vi "高压板校正命令.vi"(0 "CAN卡类型":u32(ring)=4 items=["PCI5121"=1, "PCI9810"=2, "USBCAN1"=3, "USBCAN2"=4, "PCI9820"=5, "PCI5110"=7, "CANLite(mini)"=8, "ISA9620"=9, "ISA5420"=10, "PC104CAN"=11, "DNP9810"=13, "PCI9840B"=14, "PC104C2"=15, "PCI9820I"=16, "pec9920"=18, "USBCAN_E_U"=20, "USBCAN_2E_U"=21], 1 "设备索引":u16(ring) items=["0", "1", "2", "3", "4", "5", "6", "7", "8", "9", "10", "11", "12", "13", "14", "15", ""], 2 "波特率":T4(ring)=enum."250Kbps", 3 "CAN路数":u16(ring) items=["0", "1"], 4 "Data Input":string, 5 "error in (no error)":errorcluster caption="错误输入（无错误）", 6 "滤波方式":u8(ring)=1 items=["Dual Filter", "Single Filter"], 8 "传入类型":enum16{"ASCII字符", "16进制字符"}(ring), 10 "工作方式":u8(ring) items=["Normal", "Listen Only"], 11 "校准命令":T3(ring)) -> (14 "结果":bool=TRUE, 15 "VCI_CAN_OBJ_R":T2={"ID"=0, "TimeStamp"=0, "TimeFlag"=0, "SendType"=1, "RemoteFlag"=0, "ExternFlag"=0, "DataLen"=8, 0, 0, 0, 0, 0, 0, 0, 0, 0, 0, 0} {"ID" format="%x"}, 16 "添加的数组":u8[](array[numeric]), 19 "错误输出":errorcluster)   [LabVIEW 2013]
uses:
  data/ControlCAN.dll
panel:
  out "E-U_baud":u32(ring)=393223 items=["0x060003--1000Kbps"=393219, "0x060004--800Kbps"=393220, "0x060007--500Kbps"=393223, "0x1C0008--250Kbps"=1835016, "0x1C0011--125Kbps"=1835025, "0x160023--100Kbps"=1441827, "0x1C002C--50Kbps"=1835052, "0x1600B3--20Kbps"=1441971, "0x1C00E0--10Kbps"=1835232, "0x1C01C1--5Kbps"=1835457]
  in  "等待时间（毫秒）":u32=500
  in  "times":dbl
  out "簇":T1
  out "输出簇":T2 {"ID" format="%x"}
  out "VCI_CAN_OBJ_T 2":T2
  out "子字符串":string
  in  "期望字符串":string
  in  "长度":i32
  out "VCI_CAN_OBJ_T":T2 {"ID" format="%x"}
  in  "DeviceType 5":u16(ring)=1 items=["PCI5121"=1, "PCI9810"=2, "USBCAN1"=3, "USBCAN2"=4, "PCI9820"=5, "CAN232"=6, "PCI5110"=7, "CANLite(mini)"=8, "ISA9620"=9, "ISA5420"=10, "PC104CAN"=11, "CANETE"=12, "DNP9810"=13]
  in  "CAN Channel 3":u16(ring) items=["0", "1"]
  in  "DeviceType 4":u16(ring)=1 items=["PCI5121"=1, "PCI9810"=2, "USBCAN1"=3, "USBCAN2"=4, "PCI9820"=5, "CAN232"=6, "PCI5110"=7, "CANLite(mini)"=8, "ISA9620"=9, "ISA5420"=10, "PC104CAN"=11, "CANETE"=12, "DNP9810"=13]
  in  "Accept Code":u32 format="%08x"
  in  "Mask Code":u32=4294967295 format="%08x"
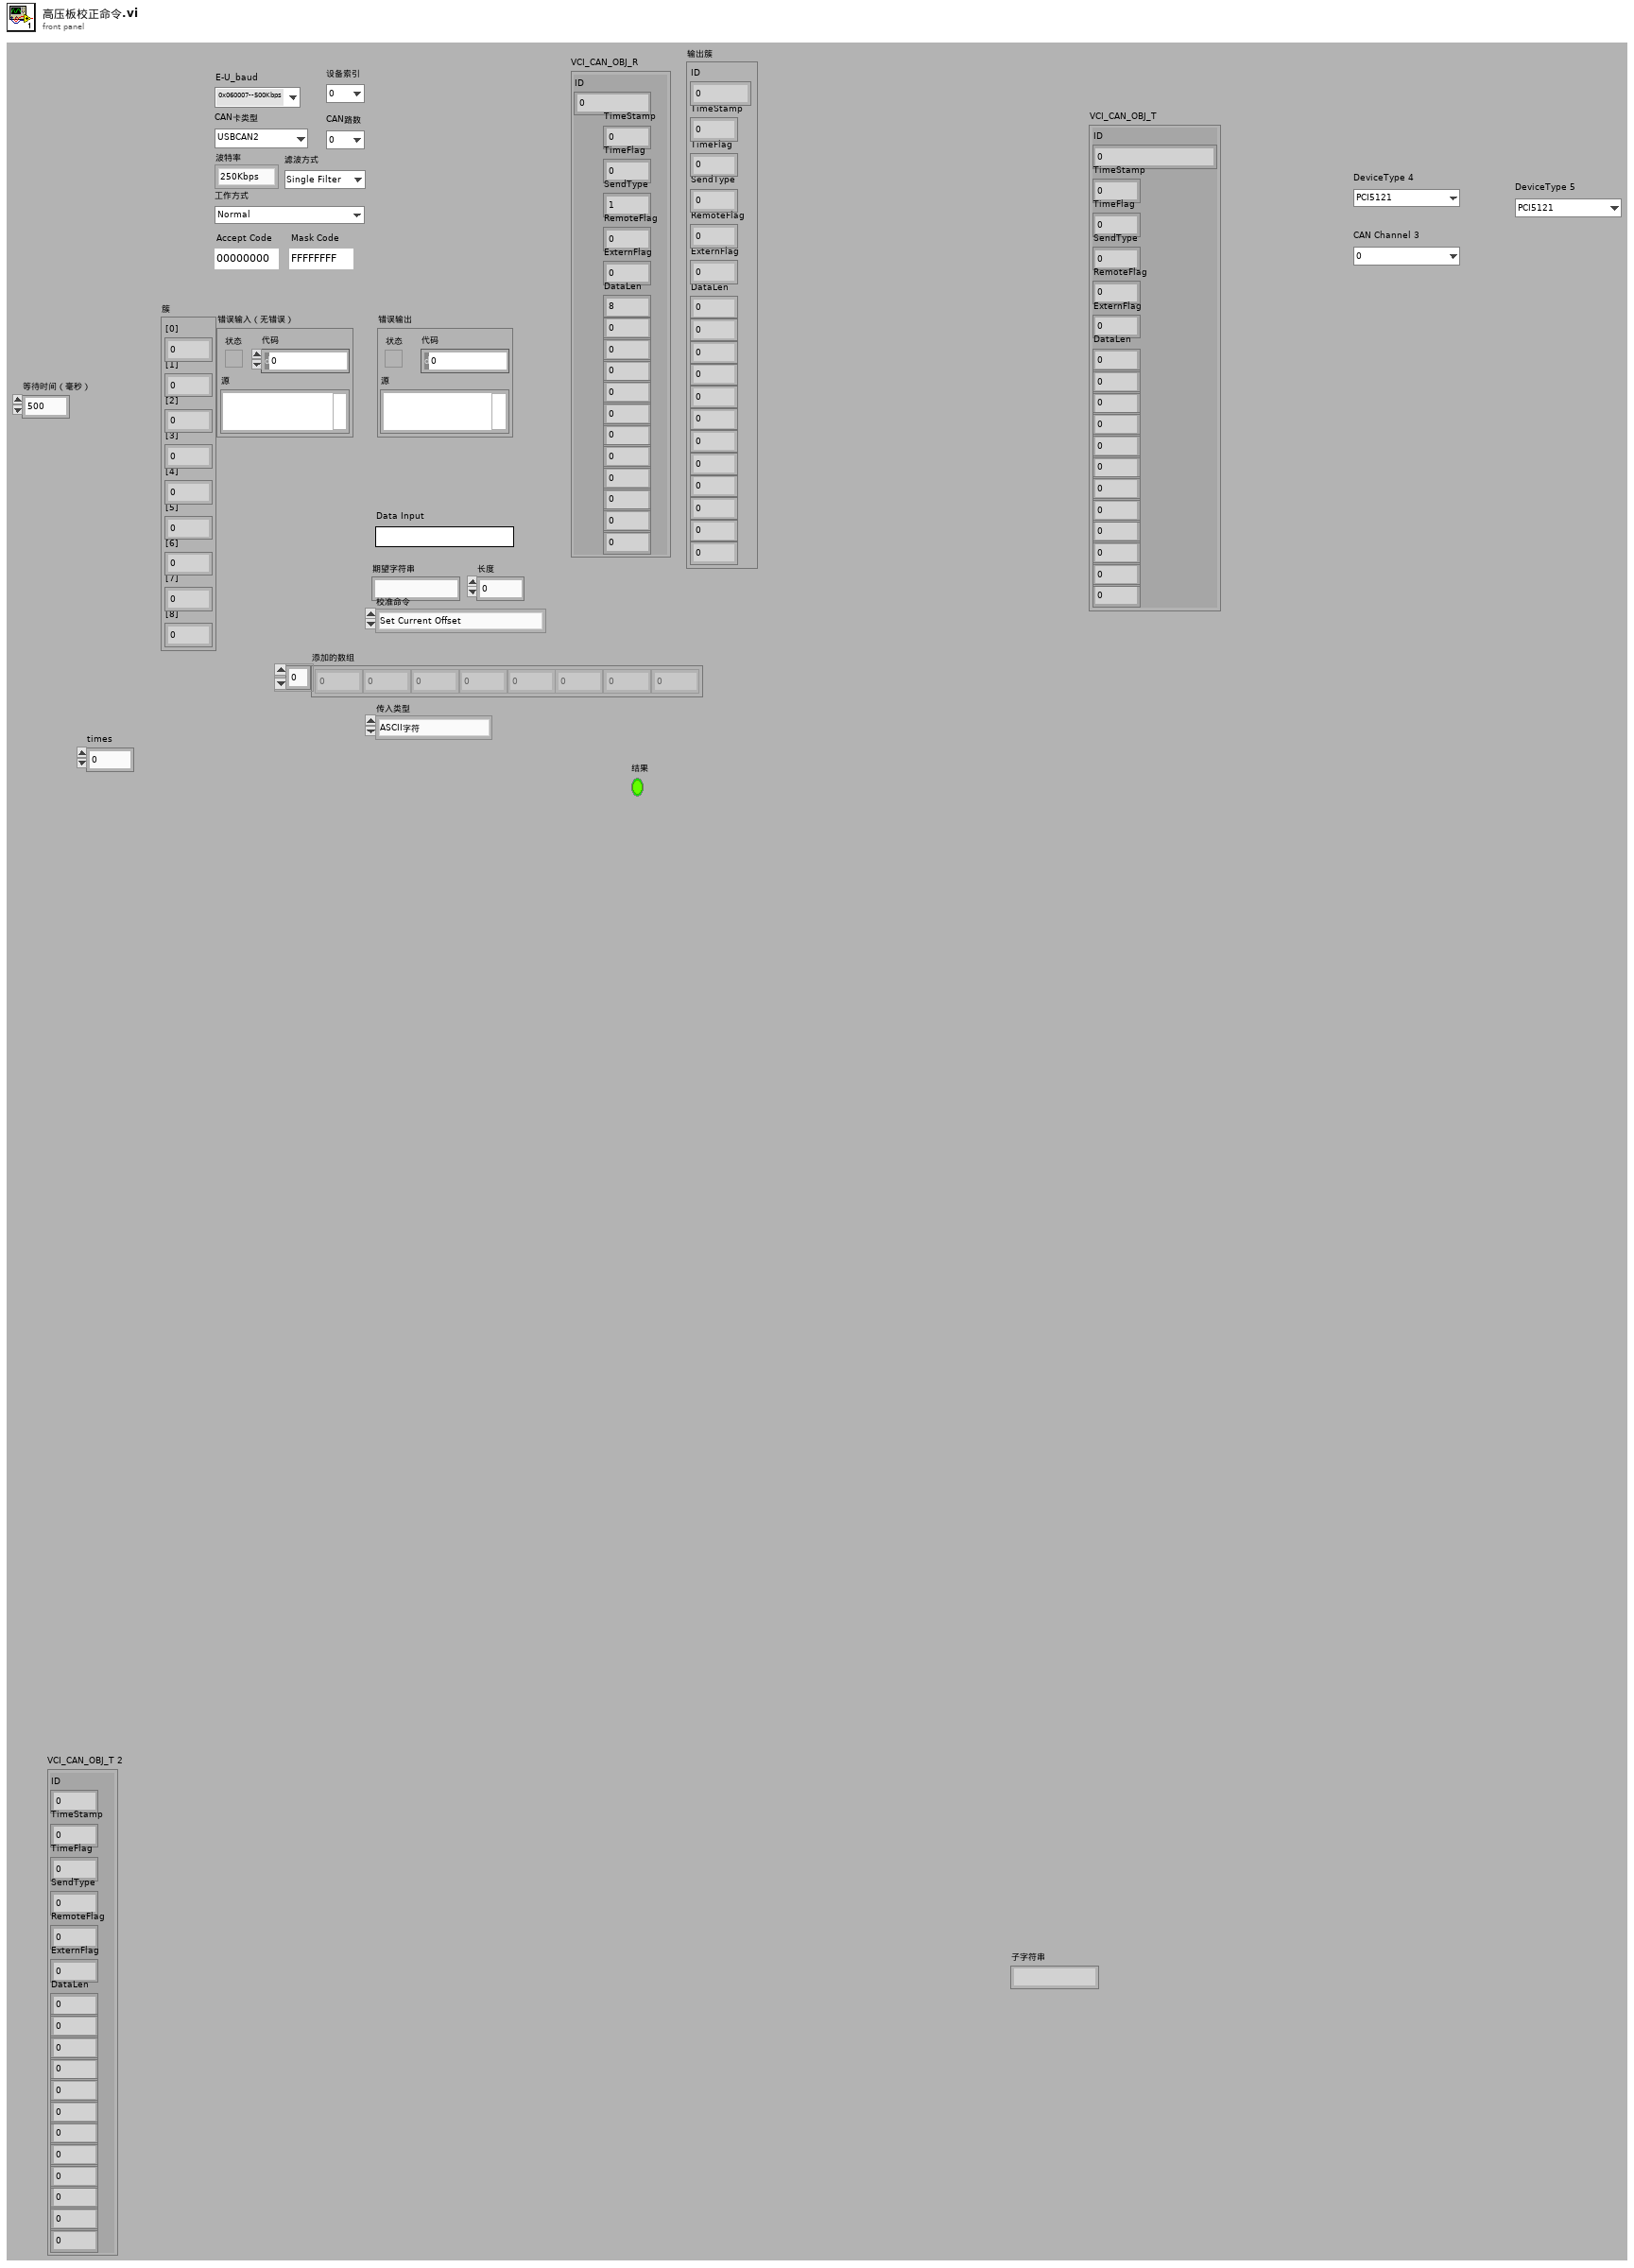
[diagram p1: front panel]
types:
  T1 = cluster{"[0]":i32, "[1]":i32, "[2]":i32, "[3]":i32, "[4]":i32, "[5]":i32, "[6]":i32, "[7]":i32, "[8]":i32}
  T2 = cluster{"ID":u32, "TimeStamp":u32, "TimeFlag":u8, "SendType":u8, "RemoteFlag":u8, "ExternFlag":u8, "DataLen":u8, u8, u8, u8, u8, u8, u8, u8, u8, u8, u8, u8}
  T3 = enum16{"Set Current Offset", "Set Current Gain 4", "Set Current Gain", "Set Volt offset", "Set Volt Gain", "Set Current Offset 3", "Set Current Gain 3", "Set Current Offset 4", "Read", "Set", "Clear", "Read_in", "Set_in", "Clear_in", "Read_out", "Set_out", "Clear_out", "参数设置", "写配置文件版本", "读配置文件版本"}
  T4 = enum16{"5Kbps", "10Kbps", "20Kbps", "40Kbps", "50Kbps", "80Kbps", "100Kbps", "125Kbps", "200Kbps", "250Kbps", "400Kbps", "500Kbps", "666Kbps", "800Kbps", "1000Kbps"}
  T5 = cluster{"[0]":u32, "[1]":u32, "[2]":u32, "[3]":u32, "[4]":u32, "[5]":u32, "[6]":u32, "[7]":u32, "[8]":u32}
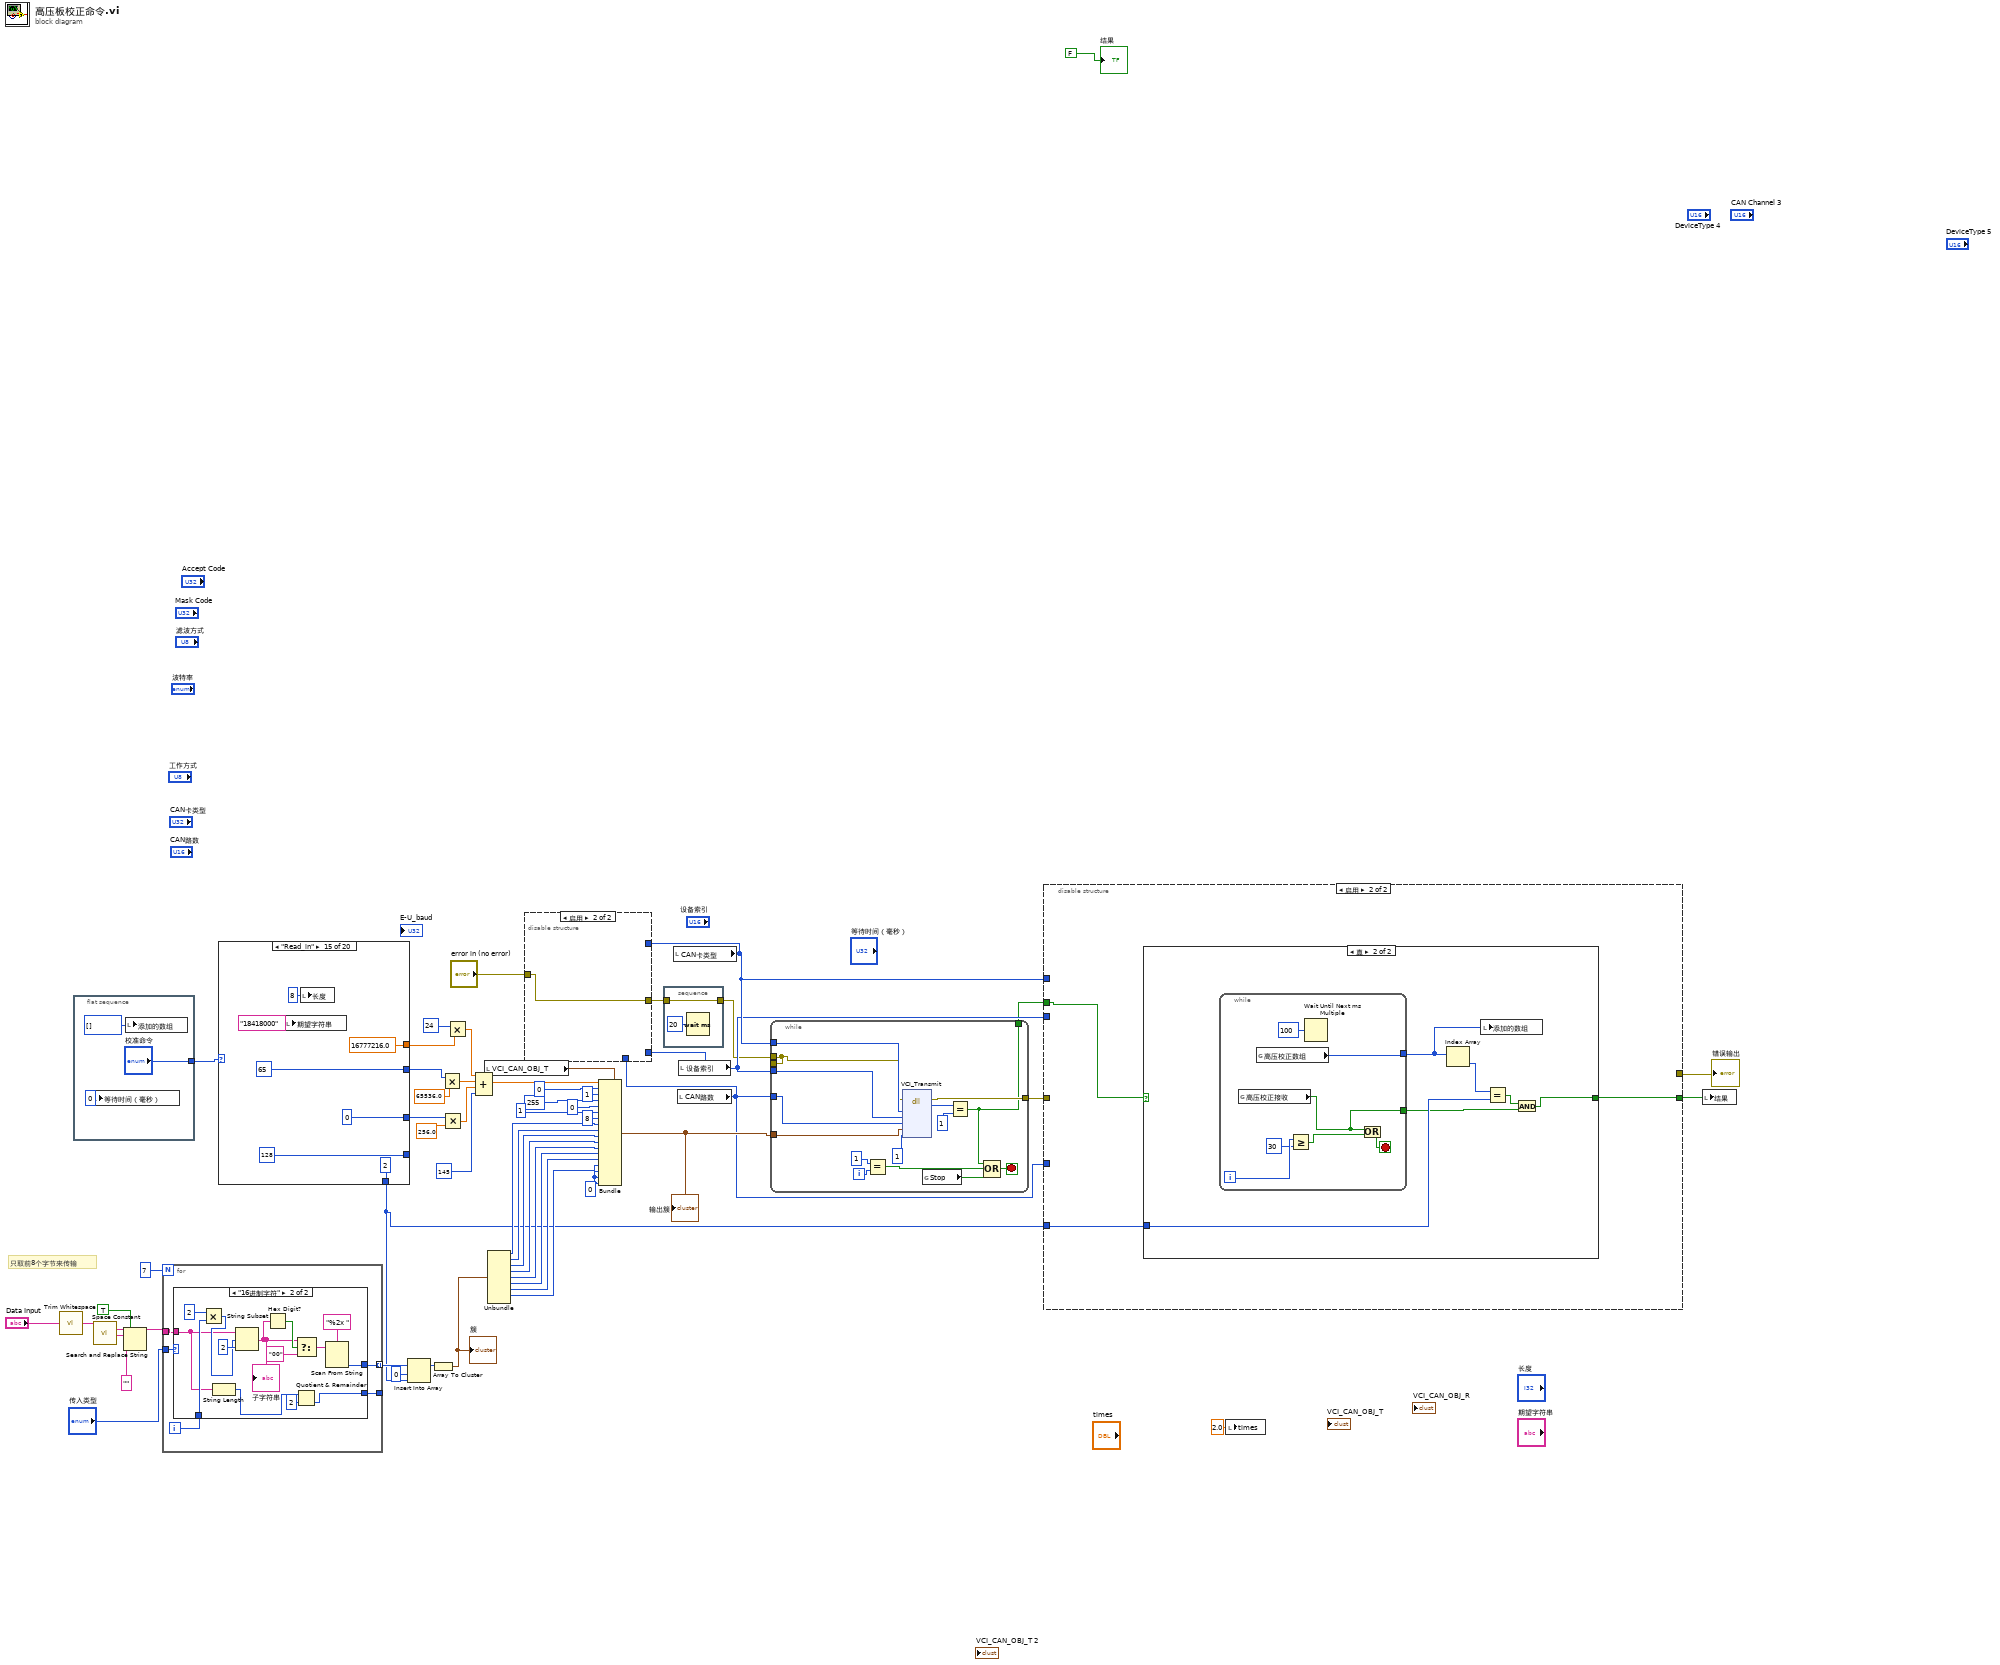
[diagram p0: block diagram]
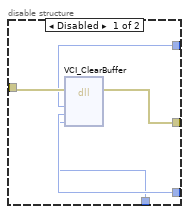
[diagram p2: hidden frame]
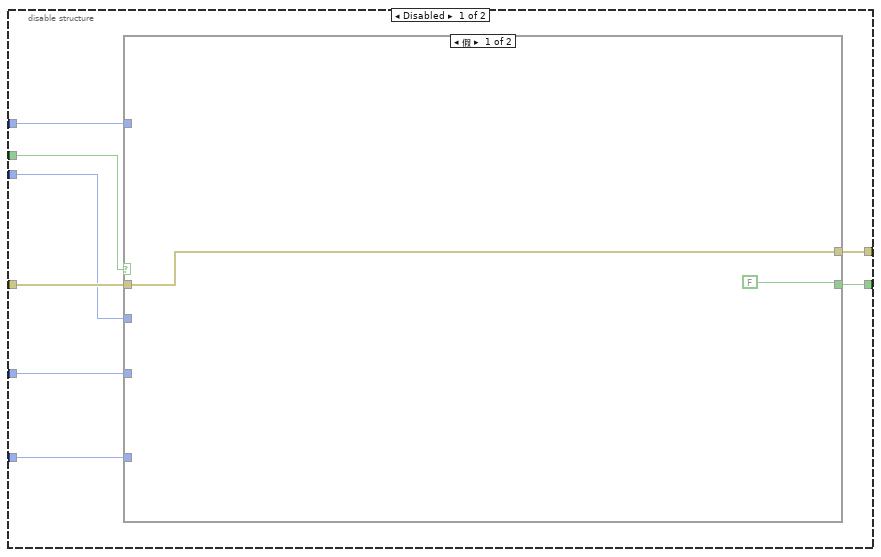
[diagram p3: hidden frame]
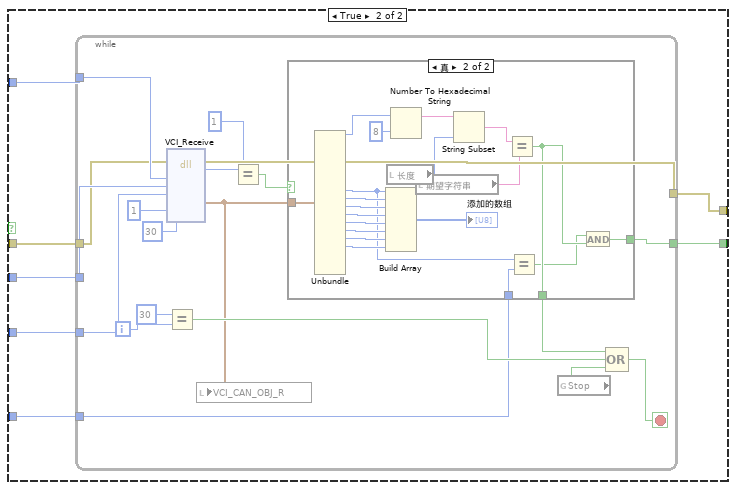
[diagram p4: hidden frame]
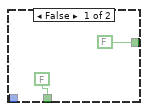
[diagram p5: hidden frame]
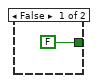
[diagram p6: hidden frame]
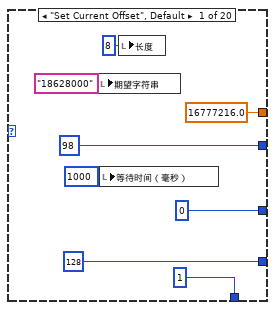
[diagram p7: hidden frame]
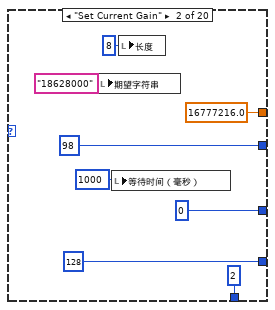
[diagram p8: hidden frame]
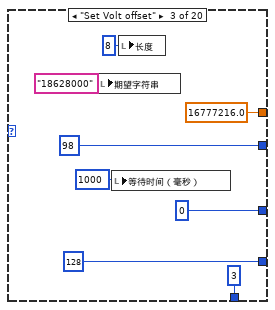
[diagram p9: hidden frame]
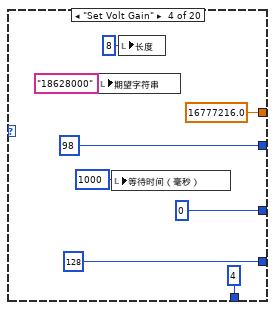
[diagram p10: hidden frame]
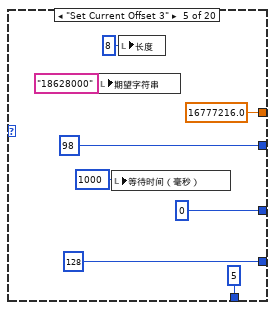
[diagram p11: hidden frame]
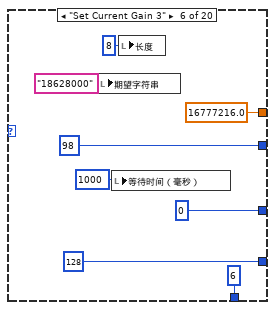
[diagram p12: hidden frame]
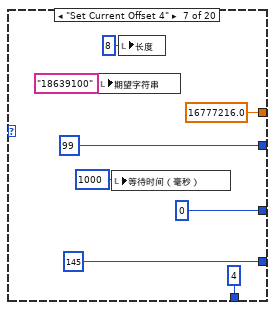
[diagram p13: hidden frame]
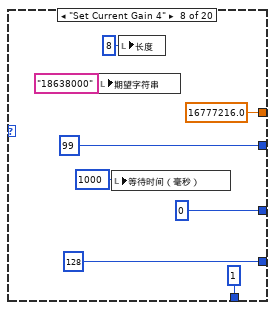
[diagram p14: hidden frame]
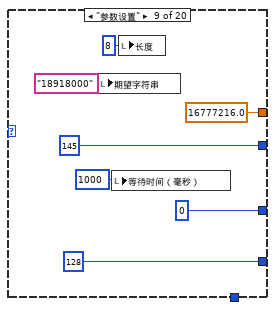
[diagram p15: hidden frame]
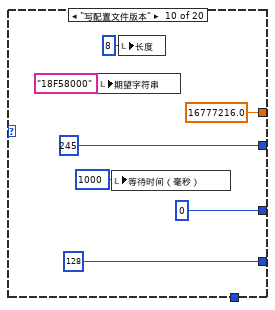
[diagram p16: hidden frame]
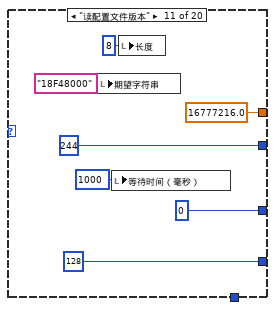
[diagram p17: hidden frame]
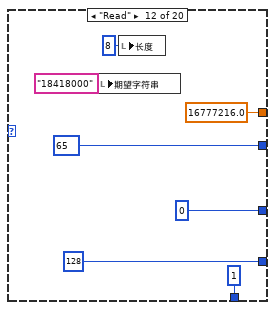
[diagram p18: hidden frame]
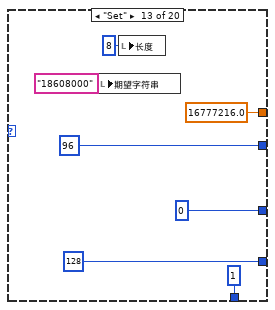
[diagram p19: hidden frame]
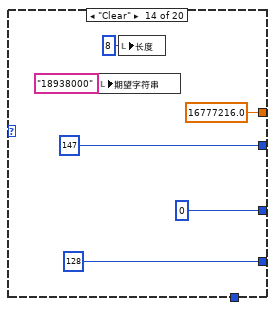
[diagram p20: hidden frame]
diagram:
  w31 = u8 0 ("元素")
  # "只取前8个字节来传输"
  n1 = call <vilib>:"Trim Whitespace.vi"("string"="Data Input") -> ("trimmed string"=w49:string)  [unwired: 1 in]
  n2 = flat-sequence {
    tunnel: ["校准命令"] -> w6
    frame #0 {
      n3 = local write "等待时间（毫秒）"(u32 0 ("等待时间（毫秒）")) -> ()
      n4 = local write "添加的数组"(u8[] [] ("添加的数组")) -> ()
    }
  }
  n5 = call <vilib>:"Space Constant.vi"() -> ("String"=w48:string)
  n6 = Search and Replace String(replace all?=TRUE ("替换全部？(F)"), input string=w49, search string=w48, replace string="" ("替换字符串(\"\")")) -> (result string=w45:string)  [unwired: 1 in, 6 out]
  n7 = for {
    N: 7 -> [_]
    tunnel: w45 -> [w60]
    tunnel: [w62] -> w53 mode=indexing
    tunnel: [w59] -> _
    tunnel: "传入类型" -> [w58]
    i -> [w61]
    n8 = case shown="\"16进制字符\"" w58 {
      tunnel: [w63 w79] -> w62
      tunnel: w61 -> [w66 w74]
      tunnel: w60 -> [w68 w72]
      tunnel: [_ w69] -> w59
      frame "ASCII字符", Default {
        n9 = String Subset(string=w68, offset (0)=w66, length (rest)=1 ("长度（剩余）")) -> (substring=w64:string)
        n10 = Type Cast(type=u8 0, x=w64) -> (*(type *) &x=w63:u8)
      }
      frame "16进制字符" {
        n11 = Multiply(x=2, y=w74) -> (x*y=w73:i32)
        n12 = String Length(string=w72) -> (length=w71:i32)
        n13 = String Subset(string=w72, offset (0)=w73, length (rest)=2 ("length (rest)")) -> (substring=w76:string)
        "子字符串" <- w76
        n14 = Hex Digit?(1:w76) -> (0:w77:bool)
        n15 = Select(t=w76, s=w77, f="00" ("t")) -> (s? t:f=w78:string)
        n16 = Quotient & Remainder(x=w71, y=2) -> (floor(x/y)=w69:i32)  [unwired: 1 out]
        n17 = Scan From String(format string="%2x ", input string=w78) -> (output 1=w79:u32)  [unwired: 2 in, 4 out]
      }
    }
  }
  n18 = case shown="\"Read_in\"" w6 {
    tunnel: [16777216.0 ("y") 16777216.0 ("y") 16777216.0 ("y") 16777216.0 ("y") 16777216.0 ("y") 16777216.0 ("y") 16777216.0 ("y") 16777216.0 ("y") 16777216.0 ("y") 16777216.0 ("y") 16777216.0 ("y") 16777216.0 ("y") 16777216.0 ("y") 16777216.0 ("y") 16777216.0 ("y") 16777216.0 ("y") 16777216.0 ("y") 16777216.0 ("y") 16777216.0 ("y") 16777216.0 ("y")] -> w43
    tunnel: [u32 98 ("x") u32 98 ("x") u32 98 ("x") u32 98 ("x") u32 98 ("x") u32 98 ("x") u32 99 ("x") u32 99 ("x") u32 145 ("x") u32 245 ("x") u32 244 ("x") u32 65 ("x") u32 96 ("x") u32 147 ("x") u32 65 ("x") u32 96 ("x") u32 149 ("x") u32 65 ("x") u32 96 ("x") u32 151 ("x")] -> w39
    tunnel: [u32 0 ("从板号") u32 0 ("从板号") u32 0 ("从板号") u32 0 ("从板号") u32 0 ("从板号") u32 0 ("从板号") u32 0 ("从板号") u32 0 ("从板号") u32 0 ("从板号") u32 0 ("从板号") u32 0 ("从板号") u32 0 ("从板号") u32 0 ("从板号") u32 0 ("从板号") u32 0 ("从板号") u32 0 ("从板号") u32 0 ("从板号") u32 0 ("从板号") u32 0 ("从板号") u32 0 ("从板号")] -> w36
    tunnel: [u32 128 ("x") u32 128 ("x") u32 128 ("x") u32 128 ("x") u32 128 ("x") u32 128 ("x") u32 145 ("x") u32 128 ("x") u32 128 ("x") u32 128 ("x") u32 128 ("x") u32 128 ("x") u32 128 ("x") u32 128 ("x") u32 128 ("x") u32 128 ("x") u32 128 ("x") u32 128 ("x") u32 128 ("x") u32 128 ("x")] -> _
    tunnel: [u32 1 ("从板号") u32 2 ("从板号") u32 3 ("从板号") u32 4 ("从板号") u32 5 ("从板号") u32 6 ("从板号") u32 4 ("从板号") u32 1 ("从板号") _ _ _ u32 1 ("从板号") u32 1 ("从板号") _ u32 2 ("从板号") u32 2 ("从板号") _ u32 3 ("从板号") u32 3 ("从板号") _] -> w3
    frame "Set Current Offset", Default {
      n19 = local write "期望字符串"("18628000" ("期望字符串")) -> ()
      n20 = local write "等待时间（毫秒）"(u32 1000 ("等待时间（毫秒）")) -> ()
      n21 = local write "长度"(8 ("长度")) -> ()
    }
    frame "Set Current Gain" {
      n22 = local write "期望字符串"("18628000" ("期望字符串")) -> ()
      n23 = local write "等待时间（毫秒）"(u32 1000 ("等待时间（毫秒）")) -> ()
      n24 = local write "长度"(8 ("长度")) -> ()
    }
    frame "Set Volt offset" {
      n25 = local write "期望字符串"("18628000" ("期望字符串")) -> ()
      n26 = local write "等待时间（毫秒）"(u32 1000 ("等待时间（毫秒）")) -> ()
      n27 = local write "长度"(8 ("长度")) -> ()
    }
    frame "Set Volt Gain" {
      n28 = local write "期望字符串"("18628000" ("期望字符串")) -> ()
      n29 = local write "等待时间（毫秒）"(u32 1000 ("等待时间（毫秒）")) -> ()
      n30 = local write "长度"(8 ("长度")) -> ()
    }
    frame "Set Current Offset 3" {
      n31 = local write "期望字符串"("18628000" ("期望字符串")) -> ()
      n32 = local write "等待时间（毫秒）"(u32 1000 ("等待时间（毫秒）")) -> ()
      n33 = local write "长度"(8 ("长度")) -> ()
    }
    frame "Set Current Gain 3" {
      n34 = local write "期望字符串"("18628000" ("期望字符串")) -> ()
      n35 = local write "等待时间（毫秒）"(u32 1000 ("等待时间（毫秒）")) -> ()
      n36 = local write "长度"(8 ("长度")) -> ()
    }
    frame "Set Current Offset 4" {
      n37 = local write "期望字符串"("18639100" ("期望字符串")) -> ()
      n38 = local write "等待时间（毫秒）"(u32 1000 ("等待时间（毫秒）")) -> ()
      n39 = local write "长度"(8 ("长度")) -> ()
    }
    frame "Set Current Gain 4" {
      n40 = local write "期望字符串"("18638000" ("期望字符串")) -> ()
      n41 = local write "等待时间（毫秒）"(u32 1000 ("等待时间（毫秒）")) -> ()
      n42 = local write "长度"(8 ("长度")) -> ()
    }
    frame "参数设置" {
      n43 = local write "期望字符串"("18918000" ("期望字符串")) -> ()
      n44 = local write "等待时间（毫秒）"(u32 1000 ("等待时间（毫秒）")) -> ()
      n45 = local write "长度"(8 ("长度")) -> ()
    }
    frame "写配置文件版本" {
      n46 = local write "期望字符串"("18F58000" ("期望字符串")) -> ()
      n47 = local write "等待时间（毫秒）"(u32 1000 ("等待时间（毫秒）")) -> ()
      n48 = local write "长度"(8 ("长度")) -> ()
    }
    frame "读配置文件版本" {
      n49 = local write "期望字符串"("18F48000" ("期望字符串")) -> ()
      n50 = local write "等待时间（毫秒）"(u32 1000 ("等待时间（毫秒）")) -> ()
      n51 = local write "长度"(8 ("长度")) -> ()
    }
    frame "Read" {
      n52 = local write "期望字符串"("18418000" ("期望字符串")) -> ()
      n53 = local write "长度"(8 ("长度")) -> ()
    }
    frame "Set" {
      n54 = local write "期望字符串"("18608000" ("期望字符串")) -> ()
      n55 = local write "长度"(8 ("长度")) -> ()
    }
    frame "Clear" {
      n56 = local write "期望字符串"("18938000" ("期望字符串")) -> ()
      n57 = local write "长度"(8 ("长度")) -> ()
    }
    frame "Read_in" {
      n58 = local write "期望字符串"("18418000" ("期望字符串")) -> ()
      n59 = local write "长度"(8 ("长度")) -> ()
    }
    frame "Set_in" {
      (unwired) u32 4 ("从板号")
      n60 = local write "期望字符串"("18608000" ("期望字符串")) -> ()
      n61 = local write "长度"(8 ("长度")) -> ()
    }
    frame "Clear_in" {
      n62 = local write "期望字符串"("18958000" ("期望字符串")) -> ()
      n63 = local write "长度"(8 ("长度")) -> ()
    }
    frame "Read_out" {
      n64 = local write "期望字符串"("18418000" ("期望字符串")) -> ()
      n65 = local write "长度"(8 ("长度")) -> ()
    }
    frame "Set_out" {
      n66 = local write "期望字符串"("18608000" ("期望字符串")) -> ()
      n67 = local write "长度"(8 ("长度")) -> ()
    }
    frame "Clear_out" {
      n68 = local write "期望字符串"("18978000" ("期望字符串")) -> ()
      n69 = local write "长度"(8 ("长度")) -> ()
    }
  }
  n70 = Insert Into Array(array=w53, index=0 ("索引"), new element=w3) -> (w5:u32[])
  n71 = Array To Cluster(array=w5) -> (cluster=w52:T5)
  "簇" <- w52
  n72 = Multiply(x=w39, y=65536.0) -> (x*y=w38:dbl)
  n73 = Multiply(x=w36, y=256.0) -> (x*y=w35:dbl)
  n74 = Multiply(x=u32 24, y=w43) -> (x*y=w42:dbl)
  n75 = Compound Arithmetic op=ADD(w42, w38, w35, u32 145 ("x")) -> (w19:dbl)
  n76 = local read "VCI_CAN_OBJ_T"() -> (w18:T2)
  n77 = Unbundle(w52) -> ("[0]"=w30:u32, "[1]"=w29:u32, "[2]"=w28:u32, "[3]"=w27:u32, "[4]"=w26:u32, "[5]"=w25:u32, "[6]"=w24:u32, "[7]"=w23:u32)  [unwired: 1 out]
  n78 = Bundle(cluster=w18, "ID"=w19, "TimeStamp"=u8 0 ("RemoteFlag"), "TimeFlag"=u8 1, "SendType"=u8 255 ("DataLen"), "RemoteFlag"=u8 0, "ExternFlag"=u8 1, "DataLen"=u8 8, w30, w29, w28, w27, w26, w25, w24, w23, w31, w31, w31) -> (w17:T2)
  "输出簇" <- w17
  n79 = local read "CAN卡类型"() -> (w12:u32)
  n80 = local read "CAN路数"() -> (w10:u16)
  n81 = local read "设备索引"() -> (w11:u16)
  n82 = disable-structure shown="启用" {
    disable-tunnel: "error in (no error)" -> [w232 w233]
    disable-tunnel: w12 -> [w231 _]
    disable-tunnel: w11 -> [w230 _]
    disable-tunnel: w10 -> [w229 _]
    disable-tunnel: [w228 w233] -> w8
    frame Disabled {
      n83 = dll-call lib="PTH1tabs FBluewave New EnergySVN_WorkBMS_Monitor_Bnet01trunkBMS_Monitor_增加二维码dataControlCAN.dll" fn="VCI_ClearBuffer" label="VCI_Clearbuffer"(error in=w232, "DeviceType"=w231, "DeviceInd"=w230, "CANInd"=w229) -> (error out=w228:errorcluster)  [unwired: 3 in, 4 out]
    }
    frame Enabled {
    }
  }
  n84 = stacked-sequence {
    tunnel: w8 -> [w235]
    tunnel: [w235] -> w7
    frame #0 {
      n85 = Wait (ms)(milliseconds to wait=u32 20 ("等待时间（毫秒）")) -> ()  [unwired: 1 out]
    }
  }
  n86 = while {
    tunnel: w12 -> [w247]
    tunnel: w11 -> [w246]
    tunnel: w10 -> [w245]
    tunnel: w17 -> [w244]
    tunnel: [w239] -> w21
    tunnel: [w238] -> _
    tunnel: w7 -> [w238]
    tunnel: [w236] -> w2
    i -> [w243]
    stop <- w240 stop-if-true
    n87 = Equal?(x=1, y=w243) -> (x = y?=w241:bool)
    n88 = dll-call lib="PTH1tabs FBluewave New EnergySVN_WorkBMS_Monitor_Bnet01trunkBMS_Monitor_增加二维码dataControlCAN.dll" fn="VCI_Transmit"(error in=w238, "DeviceType"=w247, "DeviceInd"=w246, "CANInd"=w245, "pSend"=w244, "Len"=1) -> (error out=w239:errorcluster, "返回类型"=w249:u32)  [unwired: 4 in, 4 out]
    n89 = global read "EV03全局.vi" "Stop"() -> (w237:bool)
    n90 = Equal?(x=w249, y=u32 1) -> (x = y?=w236:bool)
    n91 = Compound Arithmetic op=OR(w236, w241, w237) -> (w240:bool)
  }
  n92 = disable-structure shown="启用" {
    disable-tunnel: [w258 w310] -> w22
    disable-tunnel: w21 -> [w257 _]
    disable-tunnel: [w256 _] -> w20
    disable-tunnel: w12 -> [w255 _]
    disable-tunnel: w11 -> [w254 _]
    disable-tunnel: w10 -> [w253 _]
    disable-tunnel: w2 -> [w252 w309]
    disable-tunnel: w3 -> [w251 w311]
    frame Disabled {
      n93 = case shown="假" w252 {
        tunnel: w255 -> [_ w267]
        tunnel: w254 -> [_ w266]
        tunnel: w253 -> [_ w265]
        tunnel: [FALSE w264] -> w258
        tunnel: w257 -> [w259 w263]
        tunnel: [w259 w262] -> w256
        tunnel: w251 -> [_ w261]
        frame False {
        }
        frame True {
          n94 = while {
            tunnel: w267 -> [w285]
            tunnel: w266 -> [w284]
            tunnel: w265 -> [w283]
            tunnel: [w273] -> w264
            tunnel: w263 -> [w278]
            tunnel: [w277] -> w262
            tunnel: w261 -> [w274]
            i -> [w282]
            stop <- w279 stop-if-true
            n95 = dll-call lib="PTH1tabs FBluewave New EnergySVN_WorkBMS_Monitor_Bnet01trunkBMS_Monitor_增加二维码dataControlCAN.dll" fn="VCI_Receive"(error in=w278, "DeviceType"=w285, "DeviceInd"=w284, "CANInd"=w283, "Len"=1, "WaitTime"=30) -> (error out=w277:errorcluster, "返回类型"=w272:u32, "VCI_CAN_OBJ_R"=w275:T2)  [unwired: 5 in, 4 out]
            n96 = Equal?(x=30, y=w282) -> (x = y?=w280:bool)
            n97 = local write "VCI_CAN_OBJ_R"(w275) -> ()
            n98 = Equal?(x=w272, y=u32 1) -> (x = y?=w268:bool)
            n99 = case shown="真" w268 {
              tunnel: w275 -> [_ w308]
              tunnel: w274 -> [_ w307]
              tunnel: [FALSE w306] -> w273
              tunnel: [FALSE w302] -> w270
              frame False {
              }
              frame True {
                n100 = Unbundle(w308) -> ("ID"=w303:u32, w290:u8, w298:u8, w297:u8, w296:u8, w295:u8, w294:u8, w293:u8, w292:u8)  [unwired: 9 out]
                n101 = Build Array(w290, w298, w297, w296, w295, w294, w293, w292) -> (→"添加的数组":u8[])
                n102 = local read "长度"() -> (w300:i32)
                n103 = Number To Hexadecimal String(1:i16 8 ("宽度(-)"), 2:w303) -> (0:w305:string)
                n104 = local read "期望字符串"() -> (w301:string)
                n105 = String Subset(string=w305, length (rest)=w300) -> (substring=w299:string)  [unwired: 1 out]
                n106 = Equal?(x=w299, y=w301) -> (x = y?=w302:bool)
                n107 = Equal?(x=w290, y=w307) -> (x = y?=w289:bool)
                n108 = And(x=w289, y=w302) -> (x .and. y?=w306:bool)
              }
            }
            n109 = global read "EV03全局.vi" "Stop"() -> (w269:bool)
            n110 = Compound Arithmetic op=OR(w270, w280, w269) -> (w279:bool)
          }
        }
      }
    }
    frame Enabled {
      n111 = case shown="真" w309 {
        tunnel: w311 -> [_ w317]
        tunnel: [FALSE w313] -> w310
        frame False {
        }
        frame True {
          n112 = while {
            tunnel: [w320] -> w315
            tunnel: [w319] -> w314
            i -> [w324]
            stop <- w321 stop-if-true
            n113 = global read "EV05全局变量1.vi" "高压校正接收"() -> (w319:bool)
            n114 = global read "EV05全局变量1.vi" "高压校正数组"() -> (w320:u8[])
            n115 = Greater Or Equal?(x=w324, y=30) -> (x >= y?=w322:bool)
            n116 = Wait Until Next ms Multiple(millisecond multiple=u32 100 ("毫秒倍数")) -> ()  [unwired: 1 out]
            n117 = Or(x=w319, y=w322) -> (x .or. y?=w321:bool)
          }
          n118 = Index Array(array=w315) -> (element=w318:u8)  [unwired: 1 in]
          n119 = local write "添加的数组"(w315) -> ()
          n120 = Equal?(x=w318, y=w317) -> (x = y?=w316:bool)
          n121 = And(x=w316, y=w314) -> (x .and. y?=w313:bool)
        }
      }
    }
  }
  "错误输出" <- w20
  n122 = local write "times"(2.0 ("times")) -> ()
  n123 = local write "结果"(w22) -> ()
  "结果" <- FALSE ("CAN 操作结果")
